vi "cRIO_8maze_controls_v3.vi"() -> ()   [LabVIEW 2019]
panel:
  in  "Initialize":bool=TRUE
  in  "Air puff time":u32=1000
  in  "MD time (ms)":i32=2000
  out "Direction array":bool[](array[boolean])=[TRUE, FALSE, FALSE, TRUE, FALSE, TRUE, TRUE, FALSE, TRUE, FALSE, FALSE, TRUE, FALSE, TRUE, FALSE, FALSE, TRUE, FALSE, TRUE, TRUE, FALSE, TRUE, FALSE, FALSE, TRUE, FALSE, TRUE, TRUE, FALSE, TRUE, FALSE, FALSE, TRUE, FALSE, TRUE, TRUE, FALSE, TRUE, FALSE, FALSE, TRUE, FALSE, TRUE, TRUE, FALSE, TRUE, FALSE, FALSE, TRUE]
  out "Seq update":i32
  in  "Loop seq.":dbl
  out "All BBR":bool
  out "BB3_R":bool
  out "BB2_R":bool
  out "BB1_R":bool
  out "All BBL":bool
  out "BB3_L":bool
  out "BB2_L":bool
  out "BB1_L":bool
  out "Right":bool=TRUE
  in  "Sound":bool
  in  "AIR":bool
  out "Left":bool=TRUE
  in  "MD_R":bool
  in  "MD_L":bool
  in  "LED_R":bool
  in  "LED_L":bool
  in  "PWM rate":dbl[](array[numeric])=[0.1, 0.1, 0.1, 0.1]
  out "appended array":bool[](array[boolean])
  in  "PWM positions":dbl[](array[numeric])=[9.5, 4.0, 4.4, 8.6]
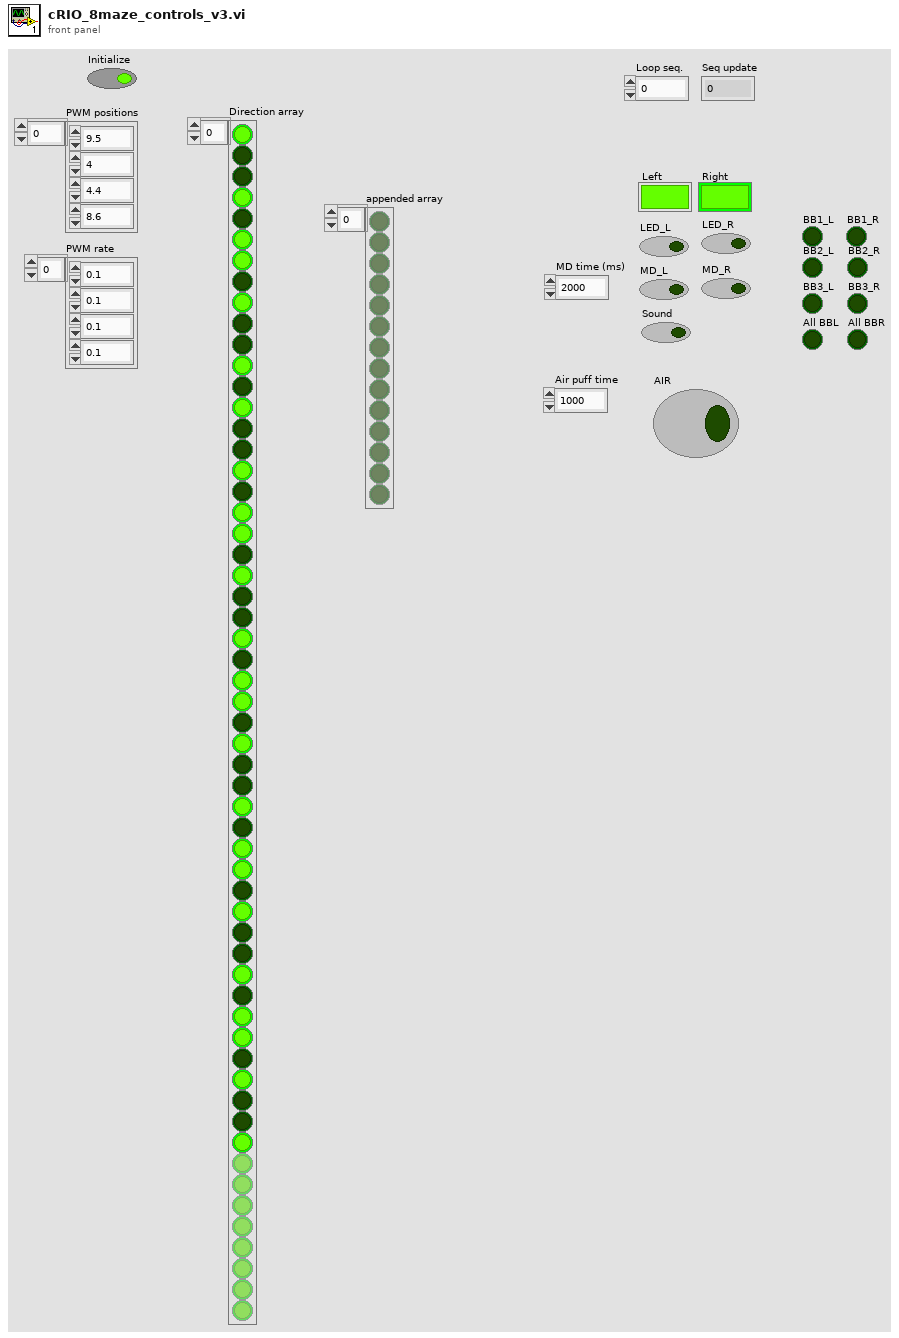
[diagram p1: front panel]
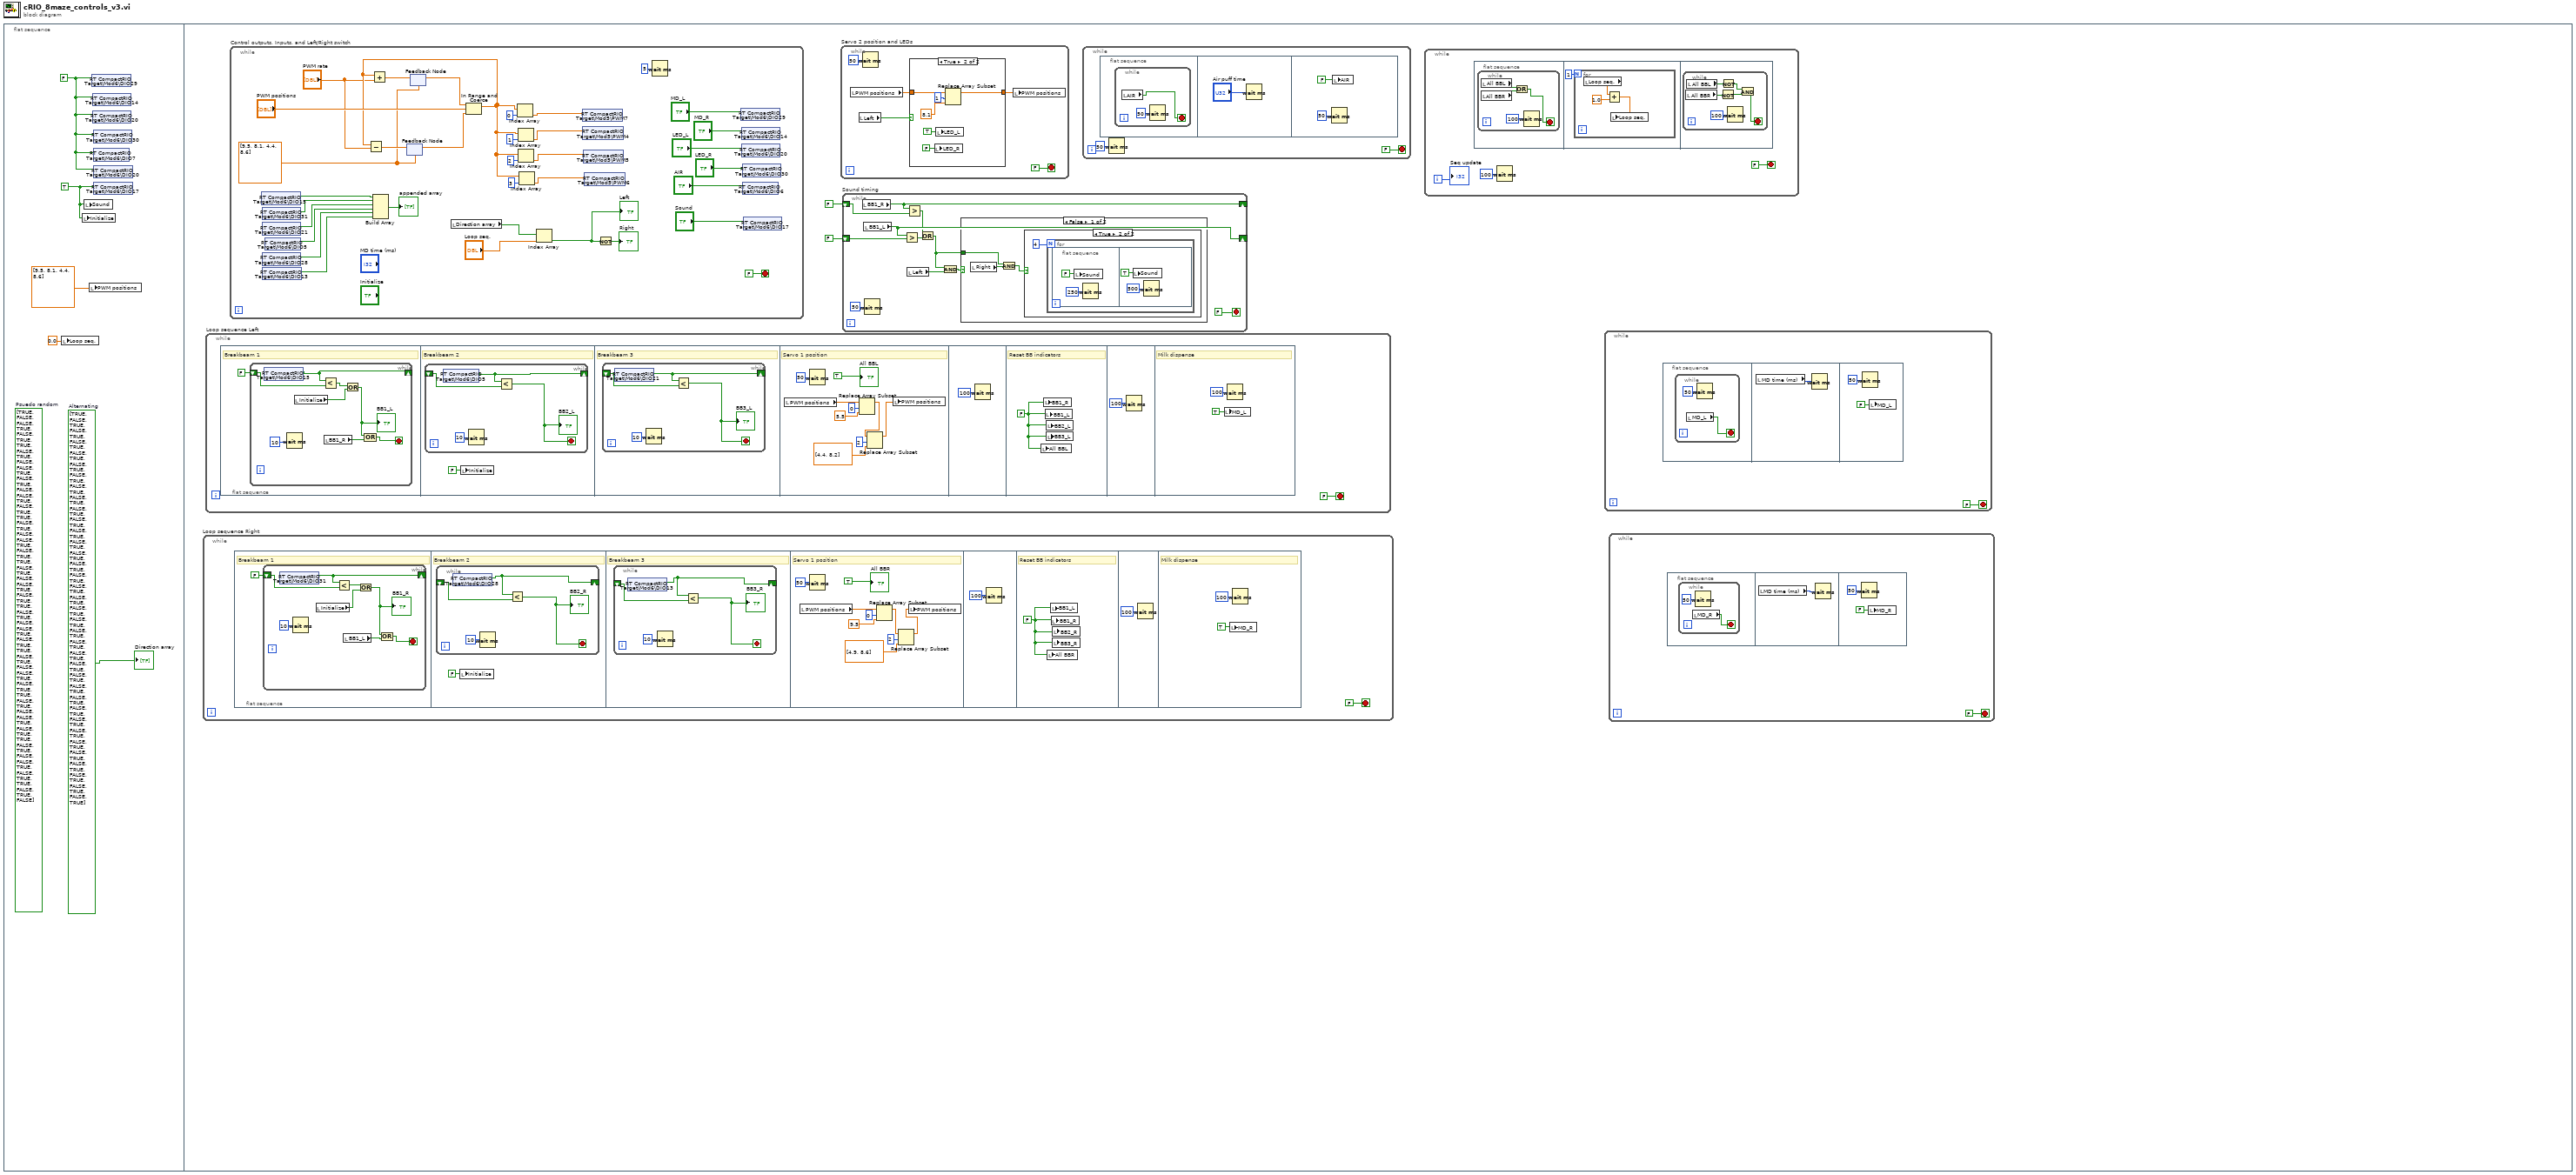
[diagram p0: block diagram]
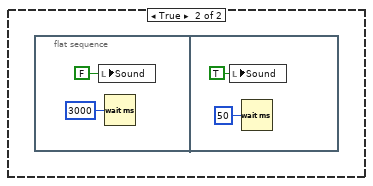
[diagram p3: hidden frame]
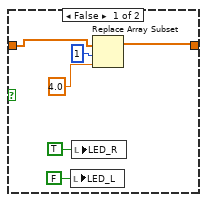
[diagram p4: hidden frame]
diagram:
  n1 = flat-sequence {
    frame #0 {
      w1 = bool[] [TRUE, FALSE, TRUE, FALSE, TRUE, FALSE, TRUE, FALSE, TRUE, FALSE, TRUE, FALSE, TRUE, FALSE, TRUE, FALSE, TRUE, FALSE, TRUE, FALSE, TRUE, FALSE, TRUE, FALSE, TRUE, FALSE, TRUE, FALSE, TRUE, FALSE, TRUE, FALSE, TRUE, FALSE, TRUE, FALSE, TRUE, FALSE, TRUE, FALSE, TRUE, FALSE, TRUE, FALSE, TRUE, FALSE, TRUE, FALSE, TRUE, FALSE, TRUE, FALSE, TRUE, FALSE, TRUE, FALSE, TRUE, FALSE, TRUE, FALSE, TRUE, FALSE, TRUE, FALSE, TRUE, FALSE, TRUE, FALSE, TRUE, FALSE, TRUE]  # Alternating
      (unwired) bool[] [TRUE, FALSE, FALSE, TRUE, FALSE, TRUE, TRUE, FALSE, TRUE, FALSE, FALSE, TRUE, FALSE, TRUE, FALSE, FALSE, TRUE, FALSE, TRUE, TRUE, FALSE, TRUE, FALSE, FALSE, TRUE, FALSE, TRUE, TRUE, FALSE, TRUE, FALSE, FALSE, TRUE, FALSE, TRUE, TRUE, FALSE, TRUE, FALSE, FALSE, TRUE, FALSE, TRUE, TRUE, FALSE, TRUE, FALSE, FALSE, TRUE, FALSE, TRUE, TRUE, FALSE, TRUE, FALSE, FALSE, TRUE, FALSE, TRUE, TRUE, FALSE, TRUE, FALSE, FALSE, TRUE, FALSE, TRUE, TRUE, FALSE, TRUE, FALSE]  # Psuedo random
      w2 = TRUE
      w5 = FALSE
      n2 = local write "Loop seq."(0.0 ("Loop seq.")) -> ()
      n3 = local write "Initialize"(w2) -> ()
      n4 = local write "Sound"(w2) -> ()
      n5 = local write "PWM positions"(dbl[] [9.5, 8.1, 4.4, 8.6]) -> ()
      n6 = shared-variable "RT CompactRIO Target\\Mod6\\DIO29"(w5) -> ()  [unwired: 1 in, 1 out]
      n7 = shared-variable "RT CompactRIO Target\\Mod6\\DIO14"(w5) -> ()  [unwired: 1 in, 1 out]
      n8 = shared-variable "RT CompactRIO Target\\Mod6\\DIO20"(w5) -> ()  [unwired: 1 in, 1 out]
      n9 = shared-variable "RT CompactRIO Target\\Mod6\\DIO30"(w5) -> ()  [unwired: 1 in, 1 out]
      n10 = shared-variable "RT CompactRIO Target\\Mod6\\DIO7"(w5) -> ()  [unwired: 1 in, 1 out]
      n11 = shared-variable "RT CompactRIO Target\\Mod6\\DIO20"(w5) -> ()  [unwired: 1 in, 1 out]
      n12 = shared-variable "RT CompactRIO Target\\Mod6\\DIO17"(w2) -> ()  [unwired: 1 in, 1 out]
      "Direction array" <- w1
    }
    frame #1 {
      n13 = while "Loop sequence Right" {
        stop <- FALSE stop-if-true
        n14 = flat-sequence {
          frame #0 {
            # "Breakbeam 1"
            n15 = while {
              shift-right: [w75] -> _
              shift-left: FALSE -> [w76]
              stop <- w72 stop-if-true
              n16 = shared-variable "RT CompactRIO Target\\Mod6\\DIO31"() -> (w75:bool)  [unwired: 1 in, 1 out]
              n17 = Wait (ms)(milliseconds to wait=u32 10) -> ()  [unwired: 1 out]
              n18 = local read "Initialize"() -> (w70:bool)
              n19 = Less?(x=w75, y=w76) -> (x < y?=w71:bool)
              n20 = local read "BB1_L"() -> (w73:bool)
              n21 = Or(x=w71, y=w70) -> (x .or. y?=w69:bool)
              "BB1_R" <- w69
              n22 = Compound Arithmetic op=OR(w69, w73) -> (w72:bool)
            }
          }
          frame #1 {
            # "Breakbeam 2"
            n23 = while {
              shift-right: [w79] -> _
              shift-left: _ -> [w81]
              stop <- w78 stop-if-true
              n24 = shared-variable "RT CompactRIO Target\\Mod6\\DIO28"() -> (w79:bool)  [unwired: 1 in, 1 out]
              n25 = Wait (ms)(milliseconds to wait=u32 10) -> ()  [unwired: 1 out]
              n26 = Less?(x=w79, y=w81) -> (x < y?=w78:bool)
              "BB2_R" <- w78
            }
            n27 = local write "Initialize"(FALSE ("Initialize")) -> ()
          }
          frame #2 {
            # "Breakbeam 3"
            n28 = while {
              shift-right: [w83] -> _
              shift-left: _ -> [w85]
              stop <- w82 stop-if-true
              n29 = shared-variable "RT CompactRIO Target\\Mod6\\DIO13"() -> (w83:bool)  [unwired: 1 in, 1 out]
              n30 = Wait (ms)(milliseconds to wait=u32 10) -> ()  [unwired: 1 out]
              n31 = Less?(x=w83, y=w85) -> (x < y?=w82:bool)
              "BB3_R" <- w82
            }
          }
          frame #3 {
            # "Servo 1 position"
            n32 = local read "PWM positions"() -> (w92:dbl[])
            n33 = Wait (ms)(milliseconds to wait=u32 50) -> ()  [unwired: 1 out]
            n34 = Replace Array Subset(array=w92, new element=9.5 ("new element/subarray"), index=0) -> (w87:dbl[])
            n35 = Replace Array Subset(array=w87, new element=dbl[] [4.9, 8.6] ("new element/subarray"), index=2) -> (w86:dbl[])
            n36 = local write "PWM positions"(w86) -> ()
            "All BBR" <- TRUE
          }
          frame #4 {
            n37 = Wait (ms)(milliseconds to wait=u32 100) -> ()  [unwired: 1 out]
          }
          frame #5 {
            w96 = FALSE
            # "Reset BB indicators"
            n38 = local write "All BBR"(w96) -> ()
            n39 = local write "BB1_L"(w96) -> ()
            n40 = local write "BB1_R"(w96) -> ()
            n41 = local write "BB2_R"(w96) -> ()
            n42 = local write "BB3_R"(w96) -> ()
          }
          frame #6 {
            n43 = Wait (ms)(milliseconds to wait=u32 100) -> ()  [unwired: 1 out]
          }
          frame #7 {
            # "Milk dispense"
            n44 = local write "MD_R"(TRUE ("MD_R")) -> ()
            n45 = Wait (ms)(milliseconds to wait=u32 100) -> ()  [unwired: 1 out]
          }
        }
      }
      n46 = while "Loop sequence Left" {
        stop <- FALSE stop-if-true
        n47 = flat-sequence {
          frame #0 {
            # "Breakbeam 1"
            n48 = while {
              shift-right: [w126] -> _
              shift-left: FALSE -> [w125]
              stop <- w122 stop-if-true
              n49 = shared-variable "RT CompactRIO Target\\Mod6\\DIO15"() -> (w126:bool)  [unwired: 1 in, 1 out]
              n50 = Wait (ms)(milliseconds to wait=u32 10) -> ()  [unwired: 1 out]
              n51 = local read "Initialize"() -> (w120:bool)
              n52 = Less?(x=w126, y=w125) -> (x < y?=w121:bool)
              n53 = local read "BB1_R"() -> (w123:bool)
              n54 = Or(x=w121, y=w120) -> (x .or. y?=w119:bool)
              "BB1_L" <- w119
              n55 = Compound Arithmetic op=OR(w119, w123) -> (w122:bool)
            }
          }
          frame #1 {
            # "Breakbeam 2"
            n56 = while {
              shift-right: [w129] -> _
              shift-left: _ -> [w131]
              stop <- w128 stop-if-true
              n57 = shared-variable "RT CompactRIO Target\\Mod6\\DIO5"() -> (w129:bool)  [unwired: 1 in, 1 out]
              n58 = Wait (ms)(milliseconds to wait=u32 10) -> ()  [unwired: 1 out]
              n59 = Less?(x=w129, y=w131) -> (x < y?=w128:bool)
              "BB2_L" <- w128
            }
            n60 = local write "Initialize"(FALSE ("Initialize")) -> ()
          }
          frame #2 {
            # "Breakbeam 3"
            n61 = while {
              shift-right: [w133] -> _
              shift-left: _ -> [w135]
              stop <- w132 stop-if-true
              n62 = shared-variable "RT CompactRIO Target\\Mod6\\DIO21"() -> (w133:bool)  [unwired: 1 in, 1 out]
              n63 = Wait (ms)(milliseconds to wait=u32 10) -> ()  [unwired: 1 out]
              n64 = Less?(x=w133, y=w135) -> (x < y?=w132:bool)
              "BB3_L" <- w132
            }
          }
          frame #3 {
            # "Servo 1 position"
            n65 = local read "PWM positions"() -> (w142:dbl[])
            n66 = Wait (ms)(milliseconds to wait=u32 50) -> ()  [unwired: 1 out]
            n67 = Replace Array Subset(array=w142, new element=5.5 ("new element/subarray"), index=0) -> (w137:dbl[])
            n68 = Replace Array Subset(array=w137, new element=dbl[] [4.4, 8.2] ("new element/subarray"), index=2) -> (w136:dbl[])
            n69 = local write "PWM positions"(w136) -> ()
            "All BBL" <- TRUE
          }
          frame #4 {
            n70 = Wait (ms)(milliseconds to wait=u32 100) -> ()  [unwired: 1 out]
          }
          frame #5 {
            w146 = FALSE
            # "Reset BB indicators"
            n71 = local write "All BBL"(w146) -> ()
            n72 = local write "BB1_R"(w146) -> ()
            n73 = local write "BB1_L"(w146) -> ()
            n74 = local write "BB2_L"(w146) -> ()
            n75 = local write "BB3_L"(w146) -> ()
          }
          frame #6 {
            n76 = Wait (ms)(milliseconds to wait=u32 100) -> ()  [unwired: 1 out]
          }
          frame #7 {
            # "Milk dispense"
            n77 = local write "MD_L"(TRUE ("MD_L")) -> ()
            n78 = Wait (ms)(milliseconds to wait=u32 100) -> ()  [unwired: 1 out]
          }
        }
      }
      n79 = while "Control outputs, Inputs, and Left/Right switch" {
        stop <- FALSE stop-if-true
        w170 = dbl[] [9.5, 8.1, 4.4, 8.6]
        n80 = shared-variable "RT CompactRIO Target\\Mod6\\DIO15"() -> (w164:bool)  [unwired: 1 in, 1 out]
        n81 = shared-variable "RT CompactRIO Target\\Mod6\\DIO31"() -> (w158:bool)  [unwired: 1 in, 1 out]
        n82 = shared-variable "RT CompactRIO Target\\Mod6\\DIO21"() -> (w159:bool)  [unwired: 1 in, 1 out]
        n83 = shared-variable "RT CompactRIO Target\\Mod6\\DIO28"() -> (w161:bool)  [unwired: 1 in, 1 out]
        n84 = shared-variable "RT CompactRIO Target\\Mod6\\DIO13"() -> (w162:bool)  [unwired: 1 in, 1 out]
        n85 = shared-variable "RT CompactRIO Target\\Mod6\\DIO5"() -> (w160:bool)  [unwired: 1 in, 1 out]
        n86 = Build Array(w164, w158, w159, w160, w161, w162) -> (→"appended array":bool[])
        n87 = feedback #1(w170) -> (w171:dbl[])
        n88 = feedback #2(w170) -> (w174:dbl[])
        n89 = local read "Direction array"() -> (w151:bool[])
        n90 = In Range and Coerce(upper limit=w174, x="PWM positions", lower limit=w171) -> (coerced(x)=w173:dbl[])  [unwired: 1 out]
        n91 = Subtract(x=w173, y="PWM rate") -> (x-y=w172:dbl[])
        n92 = Add(x=w173, y="PWM rate") -> (x+y=w175:dbl[])
        n93 = feedback-in #1(w172) -> ()
        n94 = feedback-in #2(w175) -> ()
        n95 = Index Array(array=w173, index=0) -> (element=w154:dbl)
        n96 = Index Array(array=w173, index=1) -> (element=w153:dbl)
        n97 = Index Array(array=w173, index=2) -> (element=w183:dbl)
        n98 = Index Array(array=w173, index=3) -> (element=w184:dbl)
        n99 = Index Array(array=w151, index="Loop seq.") -> (element=w152:bool)
        "Left" <- w152
        n100 = shared-variable "RT CompactRIO Target\\Mod5\\PWM7"(w154) -> ()  [unwired: 1 in, 1 out]
        n101 = shared-variable "RT CompactRIO Target\\Mod5\\PWM4"(w153) -> ()  [unwired: 1 in, 1 out]
        n102 = shared-variable "RT CompactRIO Target\\Mod5\\PWM5"(w183) -> ()  [unwired: 1 in, 1 out]
        n103 = shared-variable "RT CompactRIO Target\\Mod5\\PWM6"(w184) -> ()  [unwired: 1 in, 1 out]
        n104 = Not(x=w152) -> (.not. x?=→"Right":bool)
        n105 = Wait (ms)(milliseconds to wait=u32 5) -> ()  [unwired: 1 out]
        n106 = shared-variable "RT CompactRIO Target\\Mod6\\DIO29"("MD_L") -> ()  [unwired: 1 in, 1 out]
        n107 = shared-variable "RT CompactRIO Target\\Mod6\\DIO14"("MD_R") -> ()  [unwired: 1 in, 1 out]
        n108 = shared-variable "RT CompactRIO Target\\Mod6\\DIO20"("LED_L") -> ()  [unwired: 1 in, 1 out]
        n109 = shared-variable "RT CompactRIO Target\\Mod6\\DIO30"("LED_R") -> ()  [unwired: 1 in, 1 out]
        n110 = shared-variable "RT CompactRIO Target\\Mod6\\DIO6"("AIR") -> ()  [unwired: 1 in, 1 out]
        n111 = shared-variable "RT CompactRIO Target\\Mod6\\DIO17"("Sound") -> ()  [unwired: 1 in, 1 out]
      }
      n112 = while "Servo 2 position and LEDs" {
        stop <- FALSE stop-if-true
        n113 = local read "PWM positions"() -> (w102:dbl[])
        n114 = local read "Left"() -> (w103:bool)
        n115 = Wait (ms)(milliseconds to wait=u32 50) -> ()  [unwired: 1 out]
        n116 = case shown="True" w103 {
          tunnel: w102 -> [w108 w114]
          tunnel: [w107 w113] -> w101
          frame False {
            n117 = local write "LED_L"(FALSE ("LED_L")) -> ()
            n118 = local write "LED_R"(TRUE ("LED_R")) -> ()
            n119 = Replace Array Subset(array=w108, new element=4.0 ("new element/subarray"), index=1) -> (w107:dbl[])
          }
          frame True {
            n120 = local write "LED_R"(FALSE ("LED_R")) -> ()
            n121 = local write "LED_L"(TRUE ("LED_L")) -> ()
            n122 = Replace Array Subset(array=w114, new element=8.1 ("new element/subarray"), index=1) -> (w113:dbl[])
          }
        }
        n123 = local write "PWM positions"(w101) -> ()
      }
      n124 = while "Sound timing" {
        shift-right: [w36] -> _
        shift-left: FALSE ("BB1_L") -> [w35]
        shift-right: [w30] -> _
        shift-left: FALSE ("BB1_R") -> [w31]
        stop <- FALSE stop-if-true
        n125 = local read "BB1_R"() -> (w30:bool)
        n126 = local read "BB1_L"() -> (w36:bool)
        n127 = Wait (ms)(milliseconds to wait=u32 50) -> ()  [unwired: 1 out]
        n128 = Greater?(x=w36, y=w35) -> (0:w29:bool)
        n129 = Greater?(x=w30, y=w31) -> (0:w28:bool)
        n130 = local read "Left"() -> (w34:bool)
        n131 = Or(x=w28, y=w29) -> (x .or. y?=w27:bool)
        n132 = And(x=w27, y=w34) -> (x .and. y?=w33:bool)
        n133 = case shown="False" w33 {
          tunnel: w27 -> [w40 _]
          frame False {
            n134 = local read "Right"() -> (w39:bool)
            n135 = And(x=w40, y=w39) -> (x .and. y?=w38:bool)
            n136 = case shown="True" w38 {
              frame False {
              }
              frame True {
                n137 = for {
                  N: 4 -> [_]
                  n138 = flat-sequence {
                    frame #0 {
                      n139 = local write "Sound"(FALSE ("Sound")) -> ()
                      n140 = Wait (ms)(milliseconds to wait=u32 250) -> ()  [unwired: 1 out]
                    }
                    frame #1 {
                      n141 = local write "Sound"(TRUE ("Sound")) -> ()
                      n142 = Wait (ms)(milliseconds to wait=u32 500) -> ()  [unwired: 1 out]
                    }
                  }
                }
              }
            }
          }
          frame True {
            n143 = flat-sequence {
              frame #0 {
                n144 = local write "Sound"(FALSE ("Sound")) -> ()
                n145 = Wait (ms)(milliseconds to wait=u32 3000) -> ()  [unwired: 1 out]
              }
              frame #1 {
                n146 = local write "Sound"(TRUE ("Sound")) -> ()
                n147 = Wait (ms)(milliseconds to wait=u32 50) -> ()  [unwired: 1 out]
              }
            }
          }
        }
      }
      n148 = while {
        stop <- FALSE stop-if-true
        n149 = flat-sequence {
          frame #0 {
            n150 = while {
              stop <- w22 stop-if-true
              n151 = local read "AIR"() -> (w22:bool)
              n152 = Wait (ms)(milliseconds to wait=u32 50) -> ()  [unwired: 1 out]
            }
          }
          frame #1 {
            n153 = Wait (ms)(milliseconds to wait="Air puff time") -> ()  [unwired: 1 out]
          }
          frame #2 {
            n154 = Wait (ms)(milliseconds to wait=u32 50) -> ()  [unwired: 1 out]
            n155 = local write "AIR"(FALSE ("AIR_L")) -> ()
          }
        }
        n156 = Wait (ms)(milliseconds to wait=u32 50) -> ()  [unwired: 1 out]
      }
      n157 = while {
        i -> [w50]
        stop <- FALSE stop-if-true
        n158 = flat-sequence {
          frame #0 {
            n159 = while {
              stop <- w53 stop-if-true
              n160 = local read "All BBR"() -> (w54:bool)
              n161 = local read "All BBL"() -> (w55:bool)
              n162 = Or(x=w55, y=w54) -> (x .or. y?=w53:bool)
              n163 = Wait (ms)(milliseconds to wait=u32 100) -> ()  [unwired: 1 out]
            }
          }
          frame #1 {
            n164 = for {
              N: 1 -> [_]
              n165 = local read "Loop seq."() -> (w60:dbl)
              n166 = Add(x=w60, y=1.0) -> (x+y=w58:dbl)
              n167 = local write "Loop seq."(w58) -> ()
            }
          }
          frame #2 {
            n168 = while {
              stop <- w61 stop-if-true
              n169 = local read "All BBR"() -> (w64:bool)
              n170 = local read "All BBL"() -> (w65:bool)
              n171 = Not(x=w64) -> (.not. x?=w62:bool)
              n172 = Not(x=w65) -> (.not. x?=w63:bool)
              n173 = Wait (ms)(milliseconds to wait=u32 100) -> ()  [unwired: 1 out]
              n174 = And(x=w63, y=w62) -> (x .and. y?=w61:bool)
            }
          }
        }
        n175 = Wait (ms)(milliseconds to wait=u32 100) -> ()  [unwired: 1 out]
        "Seq update" <- w50
      }
      n176 = while {
        stop <- FALSE stop-if-true
        n177 = flat-sequence {
          frame #0 {
            n178 = while {
              stop <- w16 stop-if-true
              n179 = local read "MD_L"() -> (w16:bool)
              n180 = Wait (ms)(milliseconds to wait=u32 50) -> ()  [unwired: 1 out]
            }
          }
          frame #1 {
            n181 = local read "MD time (ms)"() -> (w17:i32)
            n182 = Wait (ms)(milliseconds to wait=w17) -> ()  [unwired: 1 out]
          }
          frame #2 {
            n183 = Wait (ms)(milliseconds to wait=u32 50) -> ()  [unwired: 1 out]
            n184 = local write "MD_L"(FALSE ("MD_L")) -> ()
          }
        }
      }
      n185 = while {
        stop <- FALSE stop-if-true
        n186 = flat-sequence {
          frame #0 {
            n187 = while {
              stop <- w10 stop-if-true
              n188 = local read "MD_R"() -> (w10:bool)
              n189 = Wait (ms)(milliseconds to wait=u32 50) -> ()  [unwired: 1 out]
            }
          }
          frame #1 {
            n190 = local read "MD time (ms)"() -> (w11:i32)
            n191 = Wait (ms)(milliseconds to wait=w11) -> ()  [unwired: 1 out]
          }
          frame #2 {
            n192 = Wait (ms)(milliseconds to wait=u32 50) -> ()  [unwired: 1 out]
            n193 = local write "MD_R"(FALSE ("MD_R")) -> ()
          }
        }
      }
    }
  }
